vi "construct.vi"(8 "error in (no error)":errorcluster, 9 "configuration name":string, 10 "load config file?":bool=TRUE, 11 "GenericPlugin in":refnum<class "TrajectoryAK101022Resonance.lvclass">) -> (0 "error out":errorcluster, 3 "GenericPlugin out":refnum<class "TrajectoryAK101022Resonance.lvclass">)   [LabVIEW 2010, in "TrajectoryAK101022Resonance.lvclass"]
uses:
  TrajectoryAK101022Resonance.lvclass
  TrajectoryMG100122GenericFPGA/TrajectoryMG100122GenericFPGA/TrajectoryMG100122GenericFPGA.lvclass
  FPGAWrapper/GenericFPGAWrapper/GenericFPGAWrapper/GenericFPGAWrapper.lvclass
  common/classes/GenericComponent/GenericComponent/GenericComponent.lvclass
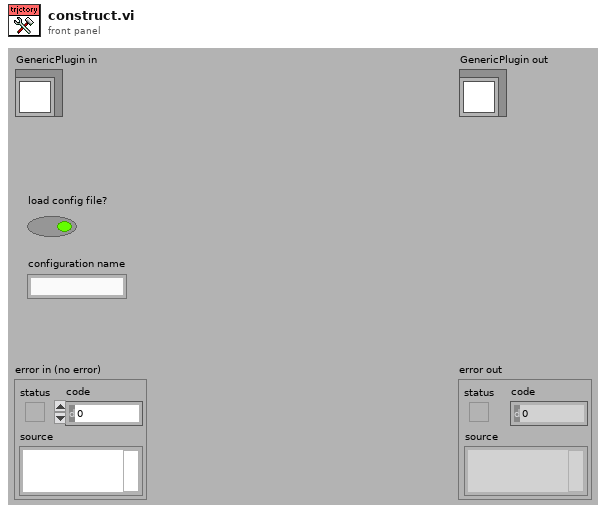
[diagram p1: front panel]
types:
  T1 = typedef "plugin_specification.ctl" = cluster{"class path":string, "configuration":string, "label":string, "settings name":string}
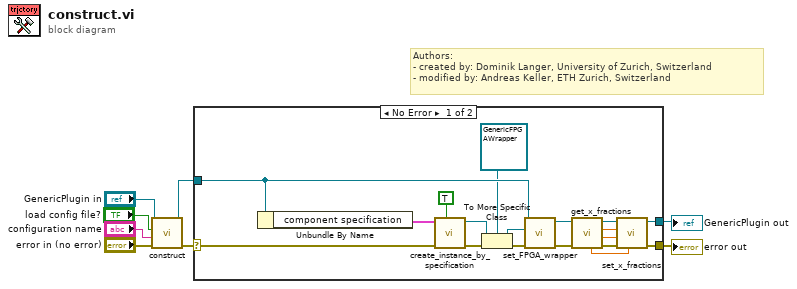
[diagram p0: block diagram]
diagram:
  # "Authors: \n- created by: Dominik Langer, University of Zurich, Switzerland\n- modified by: Andreas Keller, ETH Zurich, Switzerland"
  n1 = call-parent "construct.vi"("error in (no error)"="error in (no error)", "configuration name"="configuration name", "load config file?"="load config file?", "GenericPlugin in"="GenericPlugin in") -> ("error out"=w4:errorcluster, "GenericPlugin out"=w3:refnum<class "TrajectoryAK101022Resonance.lvclass">)  [unwired: 6 in]
  n2 = case shown="No Error" w4 {
    selector: w4 -> [w16 w27]
    tunnel: w3 -> [w17 w28]
    tunnel: [w26 w27] -> w2
    tunnel: [w25 w28] -> w1
    frame No Error {
      n3 = Unbundle By Name(w17) -> ("component specification"=w9:T1)
      n4 = call "create_instance_by_specification.vi"("call constructor?"=TRUE, "error in (no error)"=w16, "component specification"=w9) -> ("error out"=w13:errorcluster, "GenericPlugin out"=w14:refnum<class "GenericComponent.lvclass">)  [unwired: 6 in, 1 out]
      n5 = To More Specific Class(target class=refnum<class "GenericFPGAWrapper.lvclass"> refnum ("GenericFPGAWrapper.lvclass"), reference=w14, error in=w13) -> (specific class reference=w10:refnum<class "GenericFPGAWrapper.lvclass">, error out=w12:errorcluster)
      n6 = call-dynamic "set_FPGA_wrapper.vi"("error in (no error)"=w12, "GenericFPGAWrapper.lvclass"=w10, "TrajectoryMG100122GenericFPGA in"=w17) -> ("error out"=w21:errorcluster, "TrajectoryMG100122GenericFPGA out"=w20:refnum<class "TrajectoryAK101022Resonance.lvclass">)  [unwired: 7 in]
      n7 = call "get_x_fractions.vi"("error in (no error)"=w21, "TrajectoryAK101022Resonance in"=w20) -> ("error out"=w18:errorcluster, "x offset fly back fraction"=w23:dbl, "x offset fly forward fraction"=w24:dbl, "TrajectoryAK101022Resonance out"=w19:refnum<class "TrajectoryAK101022Resonance.lvclass">, "x scan segment fraction"=w22:dbl)  [unwired: 5 in]
      n8 = call-dynamic "set_x_fractions.vi"("x scan segment fraction"=w22, "error in (no error)"=w18, "x offset fly back fraction"=w23, "x offset fly forward fraction"=w24, "TrajectoryAK101022Resonance in"=w19) -> ("error out"=w26:errorcluster, "TrajectoryAK101022Resonance out"=w25:refnum<class "TrajectoryAK101022Resonance.lvclass">)  [unwired: 5 in]
    }
    frame Error {
    }
  }
  "error out" <- w2
  "GenericPlugin out" <- w1
